vi "Start.vi"(8 "error in":errorcluster, 11 "Virtual Thermometer in":refnum<class "Virtual Thermometer.lvclass">) -> (0 "error out":errorcluster, 3 "Virtual Thermometer out":refnum<class "Virtual Thermometer.lvclass">)   [LabVIEW 2024, in "Virtual Thermometer.lvclass"]
uses:
  Virtual Thermometer.lvclass
  Virtual Thermometer.lvclass/Virtual Thermometer.ctl
  Interfaces/IRunnable/IRunnable.lvclass
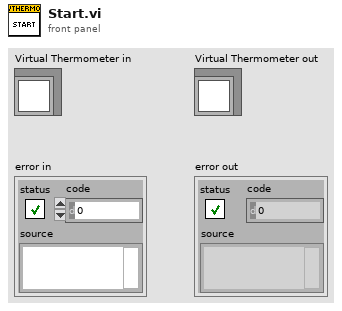
[diagram p1: front panel]
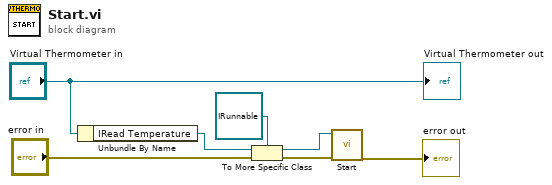
[diagram p0: block diagram]
diagram:
  n1 = Unbundle By Name("Virtual Thermometer in") -> ("IRead Temperature"=w3:refnum<class "IRead Temperature.lvclass">)
  n2 = To More Specific Class(target class=refnum<class "IRunnable.lvclass"> refnum ("IRunnable.lvclass"), reference=w3, error in="error in") -> (specific class reference=w2:refnum<class "IRunnable.lvclass">, error out=w4:errorcluster)
  n3 = call-dynamic "Start.vi"("error in"=w4, "IRunnable in"=w2) -> ("error out"=→"error out":errorcluster)  [unwired: 8 in, 1 out]
  "Virtual Thermometer out" <- "Virtual Thermometer in"
